vi "12 - Design Pattern - Flaky Delegator Design Pattern with dotNET.vi"() -> ()   [LabVIEW 2012]
uses:
  System.Windows.Forms
panel:
  in  ".NET Button -- RESET":refnum<k24>(container)
  out "Relayed event":i32
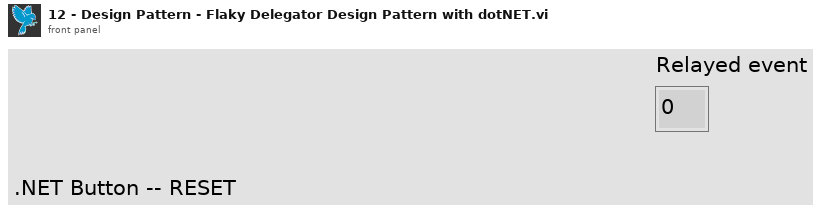
[diagram p1: front panel]
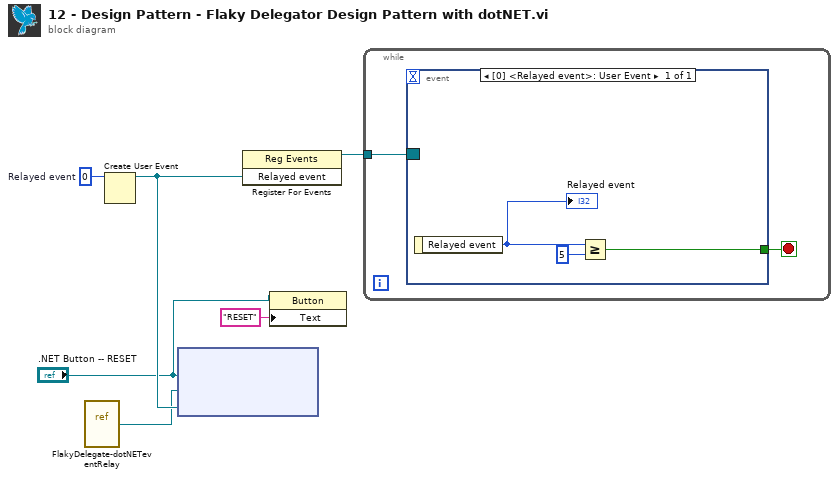
[diagram p0: block diagram]
diagram:
  w6 = 0  # Relayed event
  n1 = vi-ref "FlakyDelegate-dotNETeventRelay.vi"() -> ("vi reference"=w3:refnum<vi>)
  n2 = Create User Event(user event datatype=w6) -> (user event=w5:refnum<user-event>)  [unwired: 1 in, 1 out]
  n3 = node(".NET Button -- RESET", w3, w5) -> ()  [unwired: 2 in, 2 out]
  n4 = register-events(w5) -> (reference out=w4:refnum<event-registration>)  [unwired: 2 in, 1 out]
  n5 = property class="Button"(reference=".NET Button -- RESET", "Text"="RESET") -> ()  [unwired: 1 in, 2 out]
  n6 = while {
    tunnel: w4 -> [w7]
    stop <- w8 stop-if-true
    n7 = event shown="[0] <Relayed event>: User Event" {
      selector: w7 -> [_]
      dyn-events: _ -> [_]
      timeout: _ -> [_]
      tunnel: [w9] -> w8
      event User Event {
        n8 = event-data() -> ("Relayed event"=w11:i32)  [unwired: 1 in]
        "Relayed event" <- w11
        n9 = Greater Or Equal?(x=w11, y=5) -> (x >= y?=w9:bool)
      }
    }
  }
